vi "DequeueCmd_Cluster.vi"(8 "error in (no error)":errorcluster, 10 "Timeout (ms)":i32=-1, 11 "Queue In":T1) -> (0 "error out":errorcluster, 1 "arg[0]":string, 2 "command":string="Default", 3 "queue (dup)":T1, 4 "arguments":string[](array[string]), 5 "Data":variant)   [LabVIEW 2010]
doc: "This VI serves to dequeue a command from the queue provided to the input. The queue sorts the command from the command line arguements, which can be included after the command. The arguements are separated by a colon (:) and will be output as a string array. The VI will also handle any error that exists in the error cluster by setting the command = Error with the error code and error string message as arguments.\n\nInputs:\nQueue In - input queue (cluster)\nLog? - (bool) N/A (placeholder for future expansion)\nTimeout (ms) - (I32) timeout (in milliseconds) for the dequeue function to wait (default -1 = no timeout)\nerror in - error input cluster\n\nOutputs:\ncommand - (string) main state in the queue; this is used as the current state to be used by the case structure\ndata - (var) data enqueued with command (must be type cast in case statement)\narg[0] - (string) first argument appearing after command (if present)\narguments - command line arguments that were included with the command; separated by colon (:)\nqueue - duplicate reference for the queue\nerror out - error output cluster"
uses:
  <userlib>/Common/Queue with Cluster/TYP_Queue with Cluster Reference.ctl
panel:
  in  "Log?":bool
  # "Inputs"
  # "Outputs"
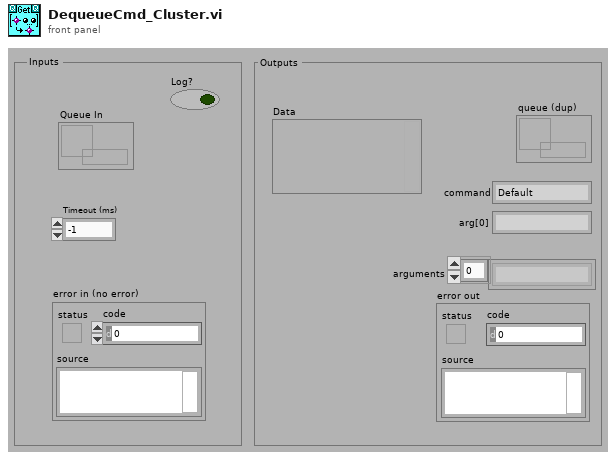
[diagram p1: front panel]
types:
  T1 = typedef "TYP_Queue with Cluster Reference.ctl" = refnum<queue>
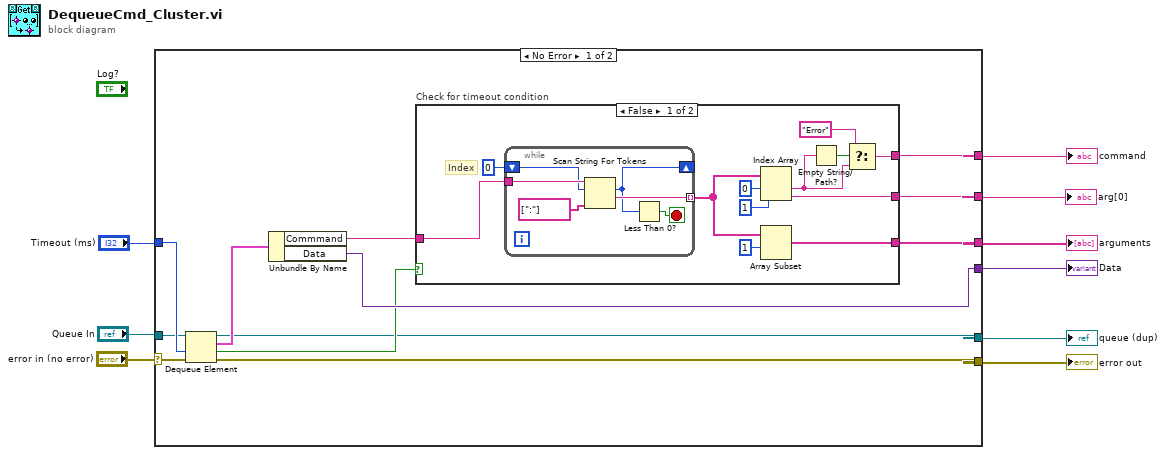
[diagram p0: block diagram]
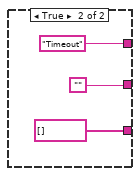
[diagram p2: hidden frame]
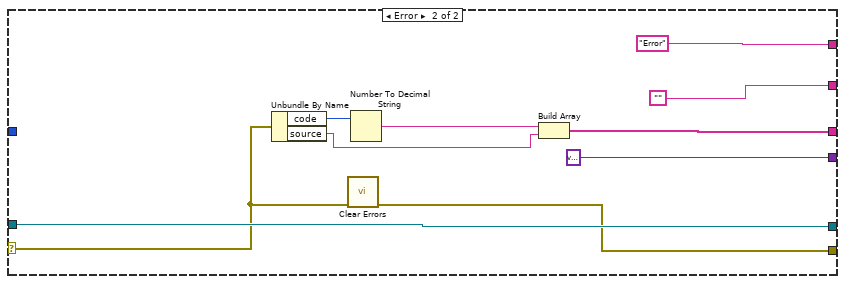
[diagram p3: hidden frame]
diagram:
  n1 = case shown="No Error" "error in (no error)" {
    selector: "error in (no error)" -> [w16 w47]
    tunnel: [w10 w46] -> w9
    tunnel: "Queue In" -> [w17 w52]
    tunnel: [w21 w49] -> w8
    tunnel: [w12 w52] -> w4
    tunnel: [w20 "Error" ("token string")] -> w7
    tunnel: [w14 variant ("Data")] -> w3
    tunnel: "Timeout (ms)" -> [w19 _]
    tunnel: [w18 ""] -> w1
    frame No Error {
      n2 = Dequeue Element(queue=w17, timeout in ms (-1)=w19, error in (no error)=w16) -> (queue out=w12:T1, element=w15:cluster{"Commmand":string, "Data":variant}, timed out?=w13:bool, error out=w10:errorcluster)
      n3 = Unbundle By Name(w15) -> ("Commmand"=w11:string, "Data"=w14:variant)
      n4 = case "Check for timeout condition" shown="False" w13 {
        tunnel: [w32 string[] []] -> w21
        tunnel: [w29 "Timeout" ("token string")] -> w20
        tunnel: [w22 ""] -> w18
        tunnel: w11 -> [w24 _]
        frame False {
          # "Index"
          n5 = while {
            tunnel: [w39] -> w25 mode=indexing
            tunnel: w24 -> [w37]
            shift-right: [w36] -> _
            shift-left: 0 ("offset past token") -> [w35]
            stop <- w38 stop-if-true
            n6 = Scan String For Tokens(6:string[] [":"] ("delimiters (\\s,\\t,\\r,\\n)"), 8:w35, 9:w37) -> (1:w39:string, 2:w36:i32)  [unwired: 3 in, 2 out]
            n7 = Less Than 0?(x=w36) -> (x < 0?=w38:bool)
          }
          n8 = Index Array(array=w25, index #1=0 ("index"), index #2=1 ("index")) -> (element #1=w27:string, element #2=w22:string)
          n9 = Array Subset(array=w25, index=1) -> (w32:string[])  [unwired: 1 in]
          n10 = Empty String/Path?(string/path=w27) -> (empty?=w28:bool)
          n11 = Select(t="Error", s=w28, f=w27) -> (s? t:f=w29:string)
        }
        frame True {
        }
      }
    }
    frame Error {
      n12 = Unbundle By Name(w47) -> ("code"=w50:i32, "source"=w45:string)
      n13 = call <vilib>:"Clear Errors.vi"("error in (no error)"=w47) -> ("error out"=w46:errorcluster)  [unwired: 6 in]
      n14 = Number To Decimal String(number=w50) -> (decimal integer string=w48:string)  [unwired: 1 in]
      n15 = Build Array(w48, w45) -> (w49:string[])
    }
  }
  "error out" <- w9
  "arguments" <- w8
  "command" <- w7
  "queue (dup)" <- w4
  "Data" <- w3
  "arg[0]" <- w1
